vi "Open Device Dani.vi"(6 "Video Format":T2, 7 "Video Res":T1, 8 "error in (no error)":errorcluster, 9 "Depth Format":T3(ring), 10 "device index":i32) -> (0 "error out":errorcluster, 3 "handle":i64)   [LabVIEW 2015]
uses:
  Controls/Video Format Control.ctl
  Controls/Video Resolution Control.ctl
  TypeDefs Host/Handle Enum.ctl
  libkinect_wrapper.dll
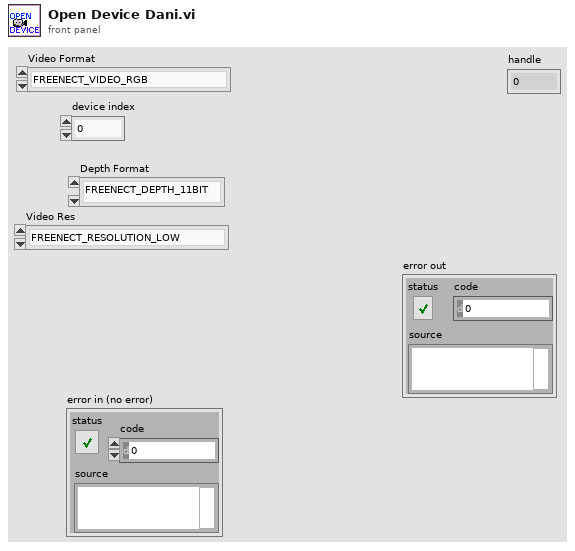
[diagram p1: front panel]
types:
  T1 = typedef "Video Resolution Control.ctl" = enum32{"FREENECT_RESOLUTION_LOW", "FREENECT_RESOLUTION_MEDIUM", "FREENECT_RESOLUTION_HIGH"}
  T2 = typedef "Video Format Control.ctl" = enum32{"FREENECT_VIDEO_RGB", "FREENECT_VIDEO_BAYER", "FREENECT_VIDEO_IR_8BIT", "FREENECT_VIDEO_IR_10BIT", "FREENECT_VIDEO_IR_10BIT_PACKED", "FREENECT_VIDEO_YUV_RGB", "FREENECT_VIDEO_YUV_RAW"}
  T3 = enum32{"FREENECT_DEPTH_11BIT", "FREENECT_DEPTH_10BIT", "FREENECT_DEPTH_11BIT_PACKED", "FREENECT_DEPTH_10BIT_PACKED", "FREENECT_DEPTH_REGISTERED", "FREENECT_DEPTH_MM"}
  T4 = typedef "Handle Enum.ctl" = enum16{"Set Handles", "Get Handles"}
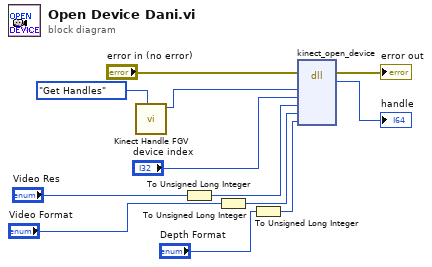
[diagram p0: block diagram]
diagram:
  n1 = call "Kinect Handle FGV.vi"("Handle Command"=Handle_Enum."Get Handles") -> ("Kinect Handle Out"=w3:i64)  [unwired: 9 in, 1 out]
  n2 = To Unsigned Long Integer(number="Video Res") -> (unsigned 32bit integer=w8:u32)
  n3 = To Unsigned Long Integer(number="Video Format") -> (unsigned 32bit integer=w7:u32)
  n4 = To Unsigned Long Integer(number="Depth Format") -> (unsigned 32bit integer=w6:u32)
  n5 = dll-call lib="libkinect_wrapper.*" fn="kinect_open_device"(error in="error in (no error)", "Context_handle"=w3, "index"="device index", "video_resolution"=w8, "video_format"=w7, "depth_format"=w6) -> (error out=→"error out":errorcluster, "handle"=→"handle":i64)  [unwired: 7 in, 1 out]
